vi "TA_Plot_3DSurface.vi"(0 "Raw TA":dbl[][](array[numeric])=array215x155[33325 elements] format="%#_8g") -> ()   [LabVIEW 2025]
uses:
  <vilib>/Math Plots/3D Math Plots/3D Surface/3D Surface Datatype/Public/Plot Helper (Vector).vi
  <vilib>/Math Plots/3D Math Plots/3D Surface/3D Surface Datatype/3D Surface Datatype.lvclass
  <vilib>/Math Plots/3D Math Plots/3D Surface/3D Surface XCtrl/3D Surface.xctl
panel:
  out "TA 3D Surface":refnum<class "3D Plot Datatype.lvclass">[](xcontrol)
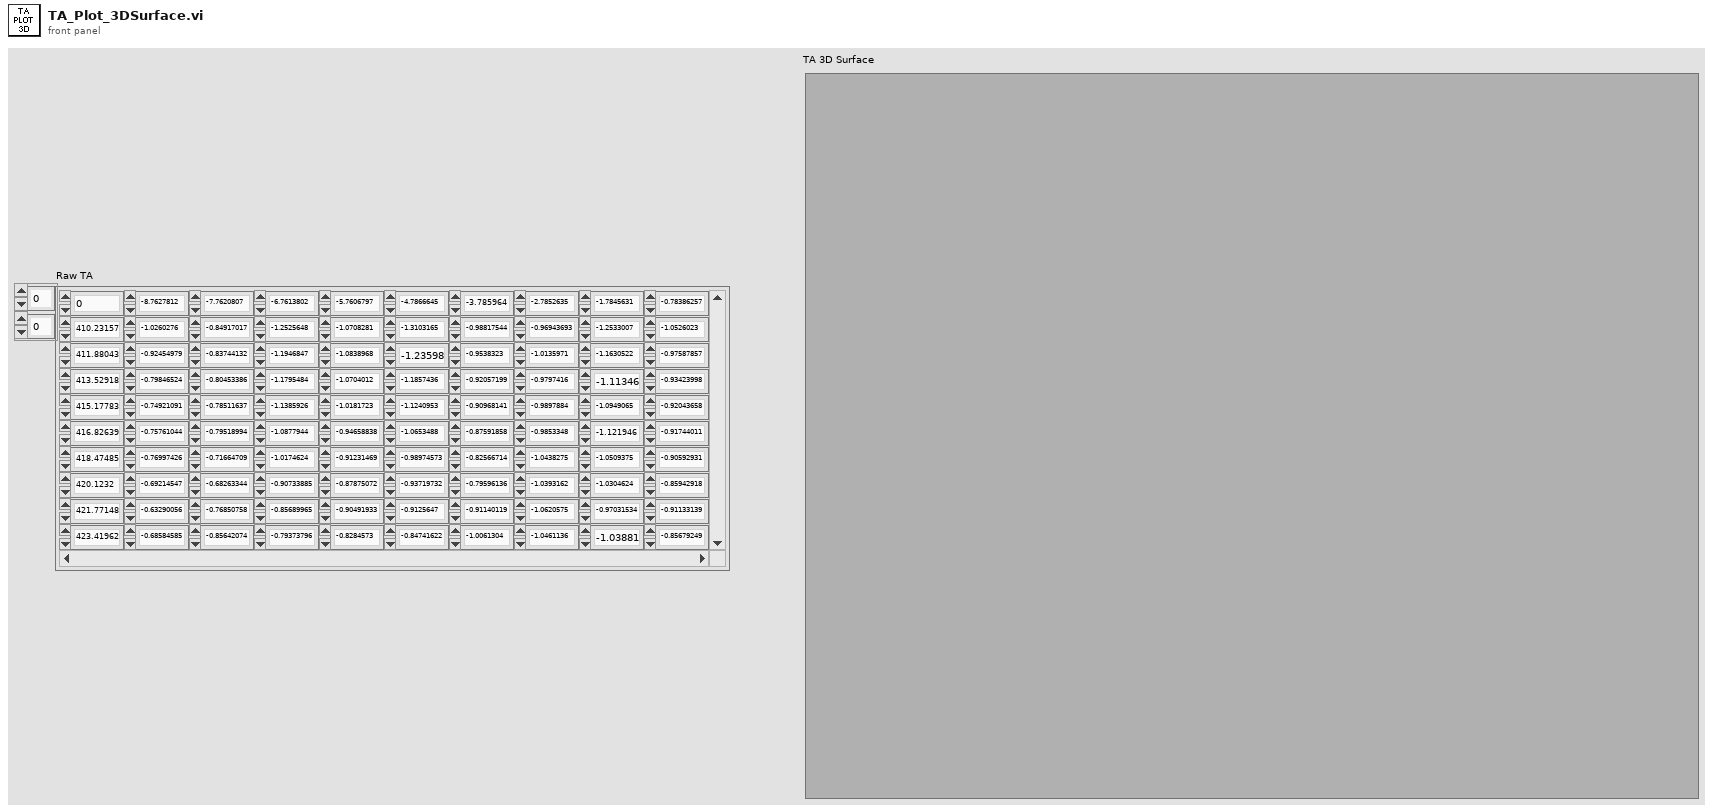
[diagram p1: front panel]
types:
  T1 = typedef "TA_DATA.ctl" = cluster{"DeltaA (mOD)":dbl[][], "Wavelength (nm)":dbl[], "Time (ps)":dbl[], "Size of DeltaA":i32[], "Size of Wavelength":i32, "Size of Time":i32}
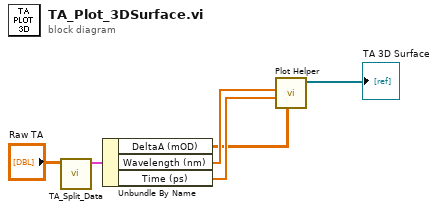
[diagram p0: block diagram]
diagram:
  n1 = call "TA_Split_Data.vi"("Raw TA"="Raw TA") -> ("TA Data"=w1:T1)  [unwired: 10 in]
  n2 = Unbundle By Name(w1) -> ("DeltaA (mOD)"=w3:dbl[][], "Wavelength (nm)"=w5:dbl[], "Time (ps)"=w4:dbl[])
  n3 = call-poly <vilib>:"Plot Helper.vi"("z matrix"=w3, "y vector"=w4, "x vector"=w5) -> ("3D Plot lvclass Array out"=→"TA 3D Surface":refnum<class "3D Plot Datatype.lvclass">[])  [unwired: 3 in, 5 out]
